vi "Get point.vi"(0 "posList":dbl[][](array[numeric]), 1 "index":dbl, 2 "currentPath":dbl[][](array[numeric])) -> (3 "Speed":dbl, 4 "Angle":dbl, 5 "check":bool, 6 "End":bool)   [LabVIEW 2022 SP3]
panel:
  out "desiredHeading":dbl
  out "heading":dbl
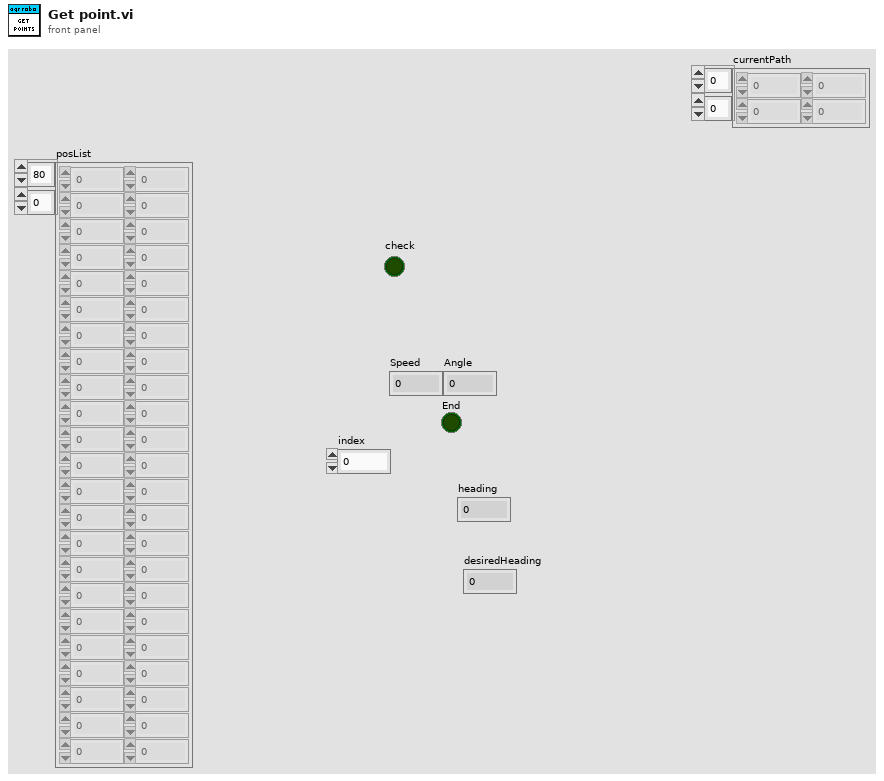
[diagram p1: front panel]
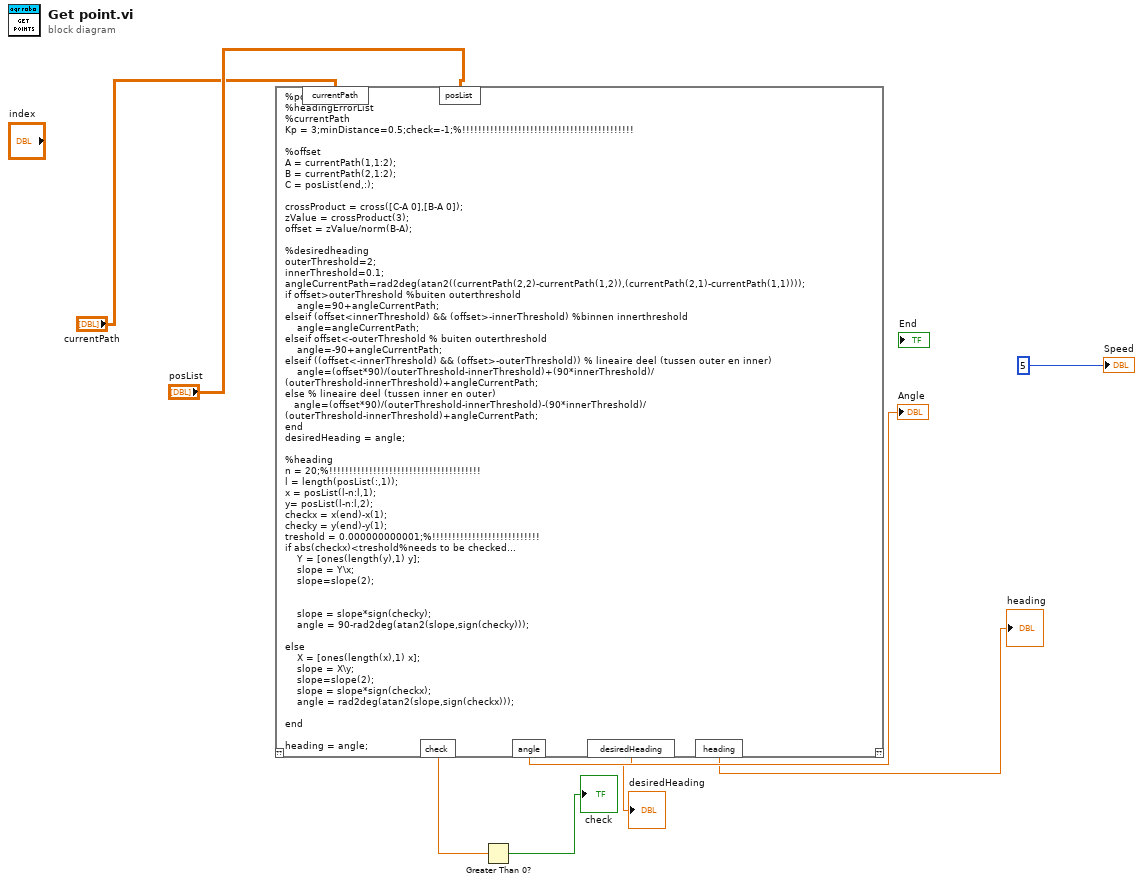
[diagram p0: block diagram]
diagram:
  n1 = script code="%posList\n%headingErrorList\n%currentPath\nKp = 3;minDistance=0.5;check=-1;%!!!!!!!!!!!!!!!!!!!!!!!!!!!!!!!!!!!!!!!!!!!\n\n%offset\nA = currentPath(1,1:2);\nB = currentPath(2,1:2);\nC = posList(end,:);\n\ncrossProduct = cross([C-A 0],[B-A 0]);\nzValue = crossProduct(3);\noffset = zValue/norm(B-A);\n\n%desiredheading\nouterThreshold=2;\ninnerThreshold=0.1;\nangleCurrentPath=rad2deg(atan2((currentPath(2,2)-currentPath(1,2)),(currentPath(2,1)-currentPath(1,1))));\nif offset>outerThreshold %buiten outerthreshold\n    angle=90+angleCurrentPath;\nelseif (offset<innerThreshold) && (offset>-innerThreshold) %binnen innerthreshold\n    angle=angleCurrentPath; \nelseif offset<-outerThreshold % buiten outerthreshold\n    angle=-90+angleCurrentPath; \nelseif ((offset<-innerThreshold) && (offset>-outerThreshold)) % lineaire deel (tussen outer en inner)\n    angle=(offset*90)/(outerThreshold-innerThreshold)+(90*innerThreshold)/(outerThreshold-innerThreshold)+angleCurrentPath;\nelse % lineaire deel (tussen inner en outer)\n   angle=(offset*90)/(outerThreshold-innerThreshold)-(90*innerThreshold)/(outerThreshold-innerThreshold)+angleCurrentPath;\nend\ndesiredHeading = angle;\n\n%heading\nn = 20;%!!!!!!!!!!!!!!!!!!!!!!!!!!!!!!!!!!!!!!\nl = length(posList(:,1));     \nx = posList(l-n:l,1);\ny= posList(l-n:l,2);\ncheckx = x(end)-x(1);\nchecky = y(end)-y(1);\ntreshold = 0.000000000001;%!!!!!!!!!!!!!!!!!!!!!!!!!!!\nif abs(checkx)<treshold%needs to be checked...\n    Y = [ones(length(y),1) y];\n    slope = Y\\x;\n    slope=slope(2);\n\n\n    slope = slope*sign(checky);\n    angle = 90-rad2deg(atan2(slope,sign(checky)));\n\nelse\n    X = [ones(length(x),1) x];\n    slope = X\\y;\n    slope=slope(2);\n    slope = slope*sign(checkx);\n    angle = rad2deg(atan2(slope,sign(checkx)));\n\nend\n\nheading = angle;\n\n\n%k regelaar\nheadingError = wrapTo360(desiredHeading)-wrapTo360(heading);\nif headingError>180\n    headingError = -(360-headingError);\nend\nif headingError<-180\n    headingError = (headingError+360);\nend\n\nangle = Kp*63*headingError/180;\n\ndistance = norm(currentPath(end,1:2)-posList(end,1:2));\nif distance<minDistance\n    check = 1;\nend\n%output : \n%angle\n%headingError\n%check"("posList"="posList", "currentPath"="currentPath") -> ("angle"=→"Angle":dbl, "desiredHeading"=→"desiredHeading":dbl, "heading"=→"heading":dbl, "check"=w3:dbl)  [unwired: 1 in, 1 out]
  n2 = Greater Than 0?(x=w3) -> (x > 0?=→"check":bool)
  "Speed" <- 5
